vi "Update-timing-led.vi"(8 "error in (no error)":errorcluster, 11 "Module status in":T1) -> (0 "error out":errorcluster, 3 "Module status":T1)   [LabVIEW 2013, in "CameraVision.lvlib" / "CV-UI.lvclass"]
uses:
  CV-UI.lvclass
  Status-overview.ctl
  Module-states.ctl
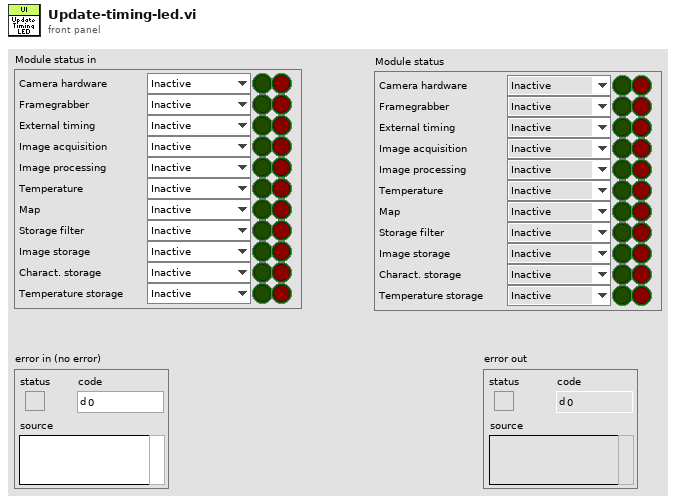
[diagram p1: front panel]
types:
  T1 = typedef "CameraVision.lvlib/CV-UI.lvclass/Status-overview.ctl" = cluster{"Camera hardware":T2, "Framegrabber":T2, "External timing":T2, "Image acquisition":T2, "Image processing ":T2, "Temperature":T2, "Map":T2, "Storage filter":T2, "Image storage":T2, "Charact. storage":T2, "Temperature storage":T2, "Camera hardware G":bool, "Camera hardware R":bool, "Framegrabber G":bool, "Framegrabber R":bool, "External timing G":bool, "External timing R":bool, "Image acquisition G":bool, "Image acquisition R":bool, "Image processing G":bool, "Image processing R":bool, "Temperature G":bool, "Temperature R":bool, "Map G":bool, "Map R":bool, "Storage filter G":bool, "Storage filter R":bool, "Image storage G":bool, "Image storage R":bool, "Charact storage G":bool, "Charact storage R":bool, "Temperature storage G":bool, "Temperature storage R":bool}
  T2 = typedef "CameraVision.lvlib/CV-UI.lvclass/Module-states.ctl" = enum16{"Inactive", "Active", "Data-loss", "Error", "Simulation", "Synchronizing", "Initialized", "Released"}
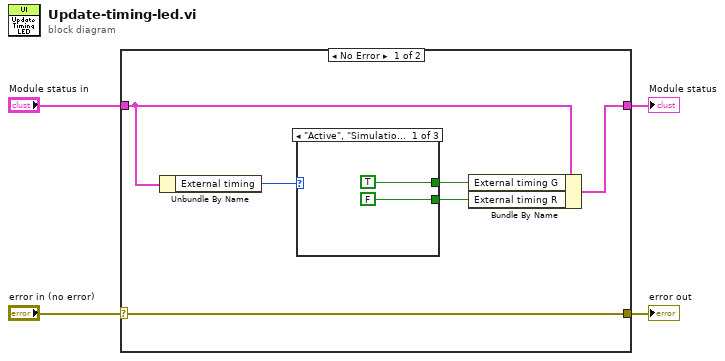
[diagram p0: block diagram]
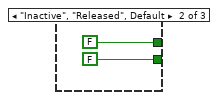
[diagram p2: hidden frame]
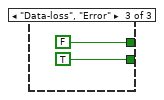
[diagram p3: hidden frame]
diagram:
  n1 = case shown="No Error" "error in (no error)" {
    selector: "error in (no error)" -> [w10 w18]
    tunnel: [w10 w18] -> w3
    tunnel: "Module status in" -> [w8 w17]
    tunnel: [w7 w17] -> w1
    frame No Error {
      n2 = Unbundle By Name(w8) -> ("External timing"=w9:T2)
      n3 = case shown="\"Active\", \"Simulation\"..\"Initialized\"" w9 {
        tunnel: [TRUE FALSE FALSE] -> w6
        tunnel: [FALSE FALSE TRUE] -> w5
        frame "Active", "Simulation".."Initialized" {
        }
        frame "Inactive", "Released", Default {
        }
        frame "Data-loss", "Error" {
        }
      }
      n4 = Bundle By Name(cluster=w8, "External timing G"=w6, "External timing R"=w5) -> (w7:T1)
    }
    frame Error {
    }
  }
  "Module status" <- w1
  "error out" <- w3
